vi "Get Key-Value Pairs.vi"(8 "error in (no error)":errorcluster, 11 "URI-Component.Query in":refnum<class "URI-Component.Query.lvclass">) -> (0 "error out":errorcluster, 2 "Query":cluster{"argument":string, "value":string}[](array[cluster]), 3 "URI-Component.Query":refnum<class "URI-Component.Query.lvclass">)   [LabVIEW 2013, in "openURI.lvlib" / "URI-Component.Query.lvclass"]
uses:
  URI-Component.Query.lvclass
  URI-Component.Query.lvclass/URI-Component.Query.ctl
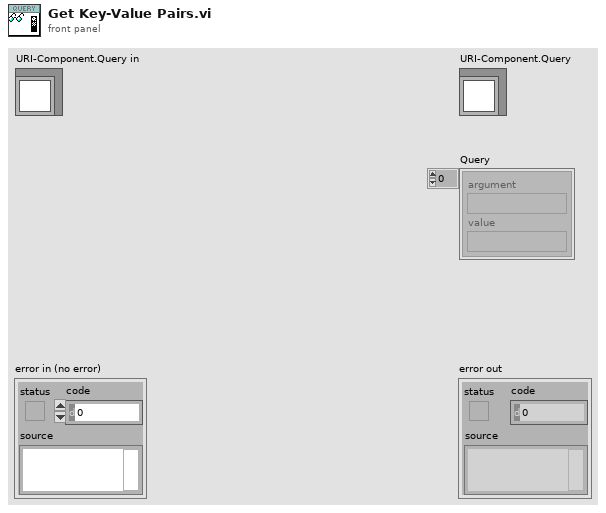
[diagram p1: front panel]
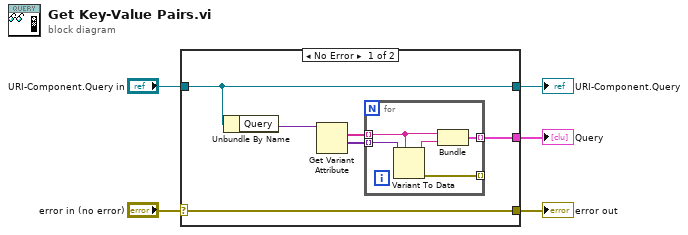
[diagram p0: block diagram]
diagram:
  n1 = case shown="No Error" "error in (no error)" {
    selector: "error in (no error)" -> [w11 w17]
    tunnel: [w11 w17] -> w4
    tunnel: [w10 w18] -> w2
    tunnel: "URI-Component.Query in" -> [w10 w18]
    tunnel: [w6 _] -> w1
    frame No Error {
      n2 = Unbundle By Name(w10) -> ("Query"=w7:variant)
      n3 = Get Variant Attribute(Variant=w7) -> (names=w8:string[], values=w9:variant[])  [unwired: 3 in, 2 out]
      n4 = for {
        tunnel: w9 -> [w16] mode=indexing
        tunnel: w8 -> [w15] mode=indexing
        tunnel: [w13] -> w6 mode=indexing
        tunnel: [w12] -> _ mode=indexing
        n5 = Variant To Data(type=w15, Variant=w16) -> (data=w14:string, error out=w12:errorcluster)  [unwired: 1 in]
        n6 = Bundle(w15, w14) -> (w13:cluster{string, string})  [unwired: 1 in]
      }
    }
    frame Error {
    }
  }
  "error out" <- w4
  "URI-Component.Query" <- w2
  "Query" <- w1
